vi "Global variables.vi"() -> ()   [LabVIEW 2019]
panel:
  in  "Ti_global":dbl
  in  "Kp_global":dbl
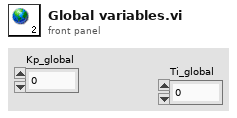
[diagram p1: front panel]
diagram:
